vi "CNT Init.vi"(9 "pConfig":T1, 10 "ChannelMask":u8, 11 "DevIndex":i32) -> (3 "function return":i32)   [LabVIEW 2010, in "usb2cnt.lvlib"]
doc: "int WINAPI CNT_Init(int DevIndex, unsigned char ChannelMask, PCNT_CONFIG pConfig);"
uses:
  usb2cnt.lvlib
  USB2XXX.dll
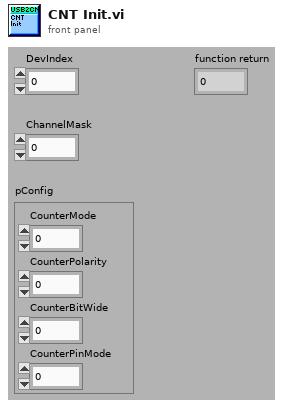
[diagram p1: front panel]
types:
  T1 = cluster{"CounterMode":u8, "CounterPolarity":u8, "CounterBitWide":u8, "CounterPinMode":u8}
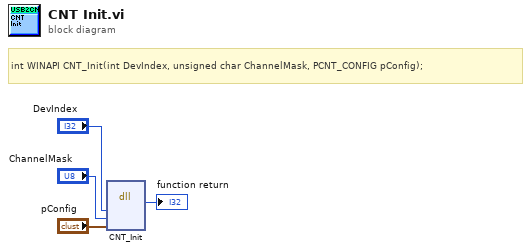
[diagram p0: block diagram]
diagram:
  # "int WINAPI CNT_Init(int DevIndex, unsigned char ChannelMask, PCNT_CONFIG pConfig);"
  n1 = dll-call lib="G:/OtherWork/USB2XXX_Example/trunk/Labview/PublicFiles/usb2cnt/USB2XXX.*" fn="CNT_Init"("DevIndex"="DevIndex", "ChannelMask"="ChannelMask", "pConfig"="pConfig") -> (→"function return":i32)  [unwired: 6 in, 2 out]
